vi "Set Steer Motors.vi"(5 "Disable":bool, 6 "PPR":dbl=1024.0, 7 "Offset Encoder Positions":dbl[](array[numeric]), 8 "Steer Control Mode":T2, 9 "Motor List":T1[](array[typedef])=[enum."Right-Front", enum."Left-Front", enum."Left-Back", enum."Right-Back"], 10 "Swerve Data":T8 {"Back Right"."Angle" scale format="%.3f"; "Back Right"."Velocity" scale=-1.0..1.0 scale format="%.1f"; "Back Left"."Angle" scale format="%.3f"; "Back Left"."Velocity" scale=-1.0..1.0 scale format="%.1f"; "Front Left"."Angle" scale format="%.3f"; "Front Left"."Velocity" scale=-1.0..1.0 scale format="%.1f"; "Front Right"."Angle" scale format="%.3f"; "Front Right"."Velocity" scale=-1.0..1.0 scale format="%.1f"}, 11 "Steer Refs":T3[](array[typedef])) -> (1 "Encoder Counts Out":dbl[](array[numeric]), 3 "Array Out":T3[](array[typedef]))   [LabVIEW 2023, in "TShirtWork-SwerveDrive_ACT_ts.lvlib"]
uses:
  TShirtWork-SwerveDrive_ACT_ts.lvlib
  <vilib>/Rock Robotics/WPI/ThirdParty/Phoenix-LabVIEW/Motor Controller/Controls/CTRE_Phoenix_MotorControl_ControlMode.ctl
  Type Defs/ENUM_Steer Mode Select.ctl
  <vilib>/Rock Robotics/SystemInterfaces/DIO/FPGA_DIOPWMChannel.ctl
  <vilib>/Rock Robotics/WPI/PWM/WPI_PWMDeadband.ctl
  <vilib>/Rock Robotics/WPI/MotorControl/WPI_MotorControlType.ctl
  <vilib>/Rock Robotics/SystemInterfaces/DIO/FPGA_DIOChannel.ctl
  <vilib>/Rock Robotics/WPI/MotorControl/WPI_MotorControlDeviceRef.ctl
  Shared Code/TypeDefs/ENUM_Module Position.ctl
  Shared Code/TypeDefs/Level_Velocity plus-minus 1.ctl
  Shared Code/TypeDefs/Dial_Compase heading unit circle CCW positive.ctl
  Shared Code/TypeDefs/Cluster_Module Velocity-Direction-Rotations.ctl
  Shared Code/TypeDefs/Cluster_Swerve 4 Steer and Velocity.ctl
panel:
  # "\"Front\" of Robot"
  # "Right Hand Rule"
  # "X"
  # "+CCW"
  # "Y"
  # "(0,0)"
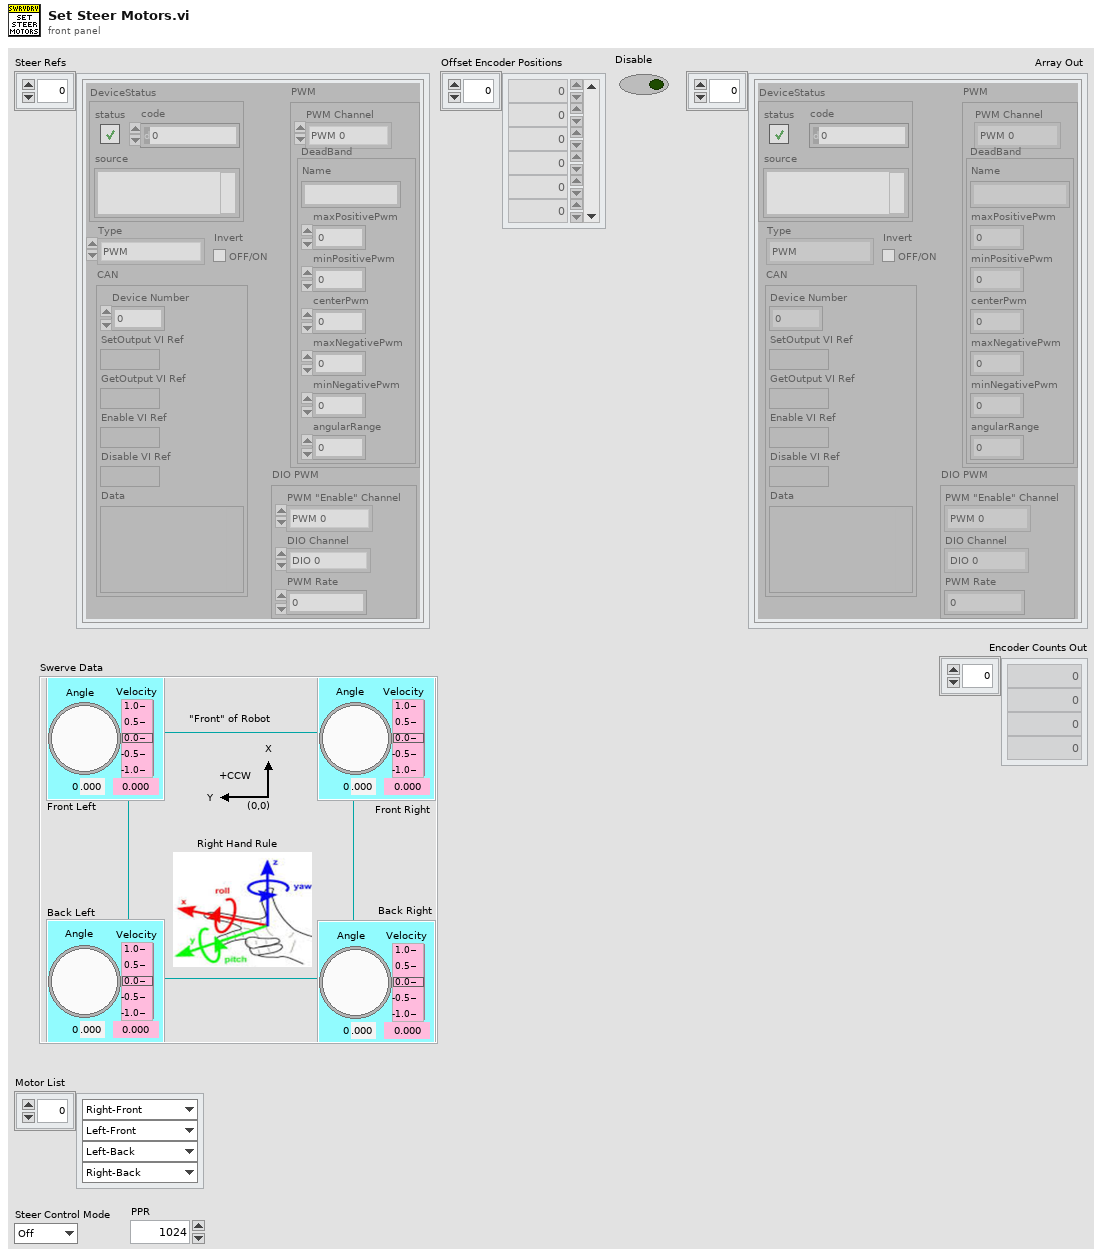
[diagram p1: front panel]
types:
  T1 = typedef "ENUM_Module Position.ctl" = enum16{"Left-Front", "Right-Front", "Left-Back", "Right-Back"}
  T2 = typedef "ENUM_Steer Mode Select.ctl" = enum16{"Off", "Hold", "Steer"}
  T3 = typedef "WPI_MotorControlDeviceRef.ctl" = cluster{"DeviceStatus":errorcluster, "Type":T4, "PWM":cluster{"PWM Channel":T5, "DeadBand":T6}, "CAN":cluster{"Device Number":u8, "SetOutput VI Ref":variant, "GetOutput VI Ref":variant, "Enable VI Ref":variant, "Disable VI Ref":variant, "Data":variant}, "Invert":bool, "DIO PWM":cluster{"PWM \"Enable\" Channel":T5, "DIOChannel":T7, "PWM Rate":dbl}}
  T4 = typedef "WPI_MotorControlType.ctl" = enum16{"PWM", "CAN", "DIO PWM"}
  T5 = typedef "FPGA_DIOPWMChannel.ctl" = enum8{"PWM 0", "PWM 1", "PWM 2", "PWM 3", "PWM 4", "PWM 5", "PWM 6", "PWM 7", "PWM 8", "PWM 9", "PWM MXP 0", "PWM MXP 1", "PWM MXP 2", "PWM MXP 3", "PWM MXP 4", "PWM MXP 5", "PWM MXP 6", "PWM MXP 7", "PWM MXP 8", "PWM MXP 9", "Invalid"}
  T6 = typedef "WPI_PWMDeadband.ctl" = cluster{"Name":string, "maxPositivePwm":i32, "minPositivePwm":i32, "centerPwm":i32, "maxNegativePwm":i32, "minNegativePwm":i32, "angularRange":u16}
  T7 = typedef "FPGA_DIOChannel.ctl" = enum8{"DIO 0", "DIO 1", "DIO 2", "DIO 3", "DIO 4", "DIO 5", "DIO 6", "DIO 7", "DIO 8", "DIO 9", "DIO MXP 0", "DIO MXP 1", "DIO MXP 2", "DIO MXP 3", "DIO MXP 4", "DIO MXP 5", "DIO MXP 6", "DIO MXP 7", "DIO MXP 8", "DIO MXP 9", "DIO MXP 10", "DIO MXP 11", "DIO MXP 12", "DIO MXP 13", "DIO MXP 14", "DIO MXP 15", "SPI Port CS1", "SPI Port CS2", "SPI Port CS3", "SPI Port MISO", "SPI Port MOSI", "Invalid"}
  T8 = typedef "Cluster_Swerve 4 Steer and Velocity.ctl" = cluster{"Front Right":T9, "Front Left":T9, "Back Left":T9, "Back Right":T9}
  T9 = typedef "Cluster_Module Velocity-Direction-Rotations.ctl" = cluster{"Velocity":T10, "Angle":T11, "Rotations Count":dbl}
  T10 = typedef "Level_Velocity plus-minus 1.ctl" = dbl
  T11 = typedef "Dial_Compase heading unit circle CCW positive.ctl" = dbl
  T12 = typedef "CTRE_Phoenix_MotorControl_ControlMode.ctl" = u16
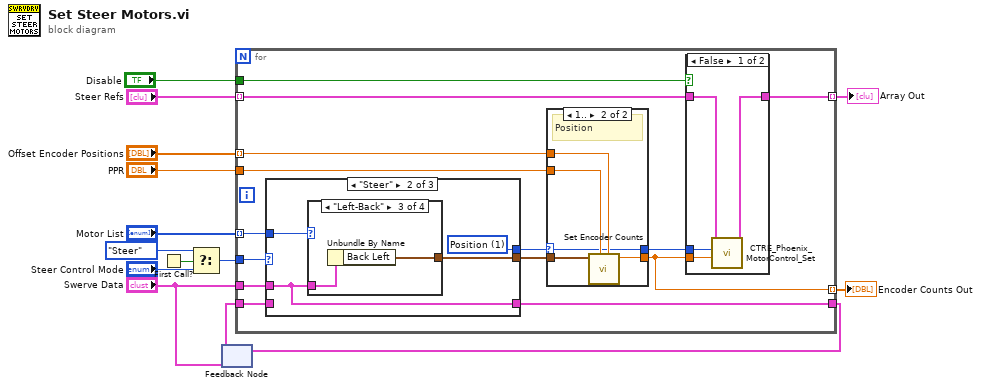
[diagram p0: block diagram]
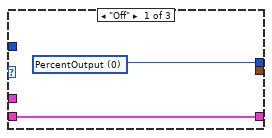
[diagram p3: hidden frame]
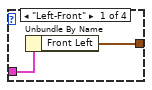
[diagram p4: hidden frame]
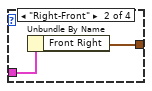
[diagram p5: hidden frame]
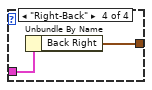
[diagram p6: hidden frame]
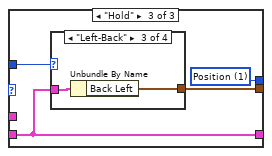
[diagram p7: hidden frame]
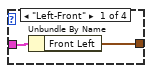
[diagram p8: hidden frame]
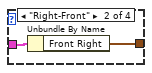
[diagram p9: hidden frame]
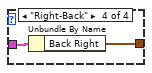
[diagram p10: hidden frame]
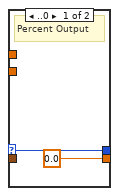
[diagram p11: hidden frame]
diagram:
  n1 = First Call?() -> (First Call?: T/F=w8:bool)
  n2 = Select(t=ENUM_Steer_Mode_Select."Steer" ("Steer Control Mode"), s=w8, f="Steer Control Mode") -> (s? t:f=w5:T2)
  n3 = feedback #1("Swerve Data") -> (w9:T8)
  n4 = for {
    tunnel: "Steer Refs" -> [w28] mode=indexing
    tunnel: "Swerve Data" -> [w25]
    tunnel: [w27] -> w14 mode=indexing
    tunnel: "Offset Encoder Positions" -> [w22] mode=indexing
    tunnel: w5 -> [w26]
    tunnel: "PPR" -> [w23]
    tunnel: "Motor List" -> [w24] mode=indexing
    tunnel: w9 -> [w20]
    tunnel: [w19] -> w3
    tunnel: [w16] -> w2 mode=indexing
    tunnel: "Disable" -> [w15]
    n5 = case shown="\"Steer\"" w26 {
      tunnel: [w35 w39 w51] -> w18
      tunnel: w25 -> [_ w36 _]
      tunnel: w24 -> [_ w38 w50]
      tunnel: [_ w37 w49] -> w21
      tunnel: w20 -> [w34 _ w48]
      tunnel: [w34 w36 w48] -> w19
      frame "Off" {
        w35 = T12 0 items=["PercentOutput"=0, "Position"=1, "Velocity"=2, "Current"=3, "Follower"=5, "MotionProfile"=6, "MotionMagic"=7, "MotionProfileArc"=10, "Disabled"=15] ("Control Mode")
      }
      frame "Steer" {
        w39 = T12 1 items=["PercentOutput"=0, "Position"=1, "Velocity"=2, "Current"=3, "Follower"=5, "MotionProfile"=6, "MotionMagic"=7, "MotionProfileArc"=10, "Disabled"=15] ("Control Mode")
        n6 = case shown="\"Left-Back\"" w38 {
          tunnel: w36 -> [w41 w43 w45 w47]
          tunnel: [w40 w42 w44 w46] -> w37
          frame "Left-Front" {
            n7 = Unbundle By Name(w41) -> ("Front Left"=w40:T9)
          }
          frame "Right-Front" {
            n8 = Unbundle By Name(w43) -> ("Front Right"=w42:T9)
          }
          frame "Left-Back" {
            n9 = Unbundle By Name(w45) -> ("Back Left"=w44:T9)
          }
          frame "Right-Back" {
            n10 = Unbundle By Name(w47) -> ("Back Right"=w46:T9)
          }
        }
      }
      frame "Hold" {
        w51 = T12 1 items=["PercentOutput"=0, "Position"=1, "Velocity"=2, "Current"=3, "Follower"=5, "MotionProfile"=6, "MotionMagic"=7, "MotionProfileArc"=10, "Disabled"=15] ("Control Mode")
        n11 = case shown="\"Left-Back\"" w50 {
          tunnel: w48 -> [w53 w55 w57 w59]
          tunnel: [w52 w54 w56 w58] -> w49
          frame "Left-Front" {
            n12 = Unbundle By Name(w53) -> ("Front Left"=w52:T9)
          }
          frame "Right-Front" {
            n13 = Unbundle By Name(w55) -> ("Front Right"=w54:T9)
          }
          frame "Left-Back" {
            n14 = Unbundle By Name(w57) -> ("Back Left"=w56:T9)
          }
          frame "Right-Back" {
            n15 = Unbundle By Name(w59) -> ("Back Right"=w58:T9)
          }
        }
      }
    }
    n16 = case shown="1.." w18 {
      selector: w18 -> [w60 w62]
      tunnel: w21 -> [_ w65]
      tunnel: w23 -> [_ w64]
      tunnel: w22 -> [_ w63]
      tunnel: [0.0 ("Encder Count Set") w66] -> w16
      tunnel: [w60 w62] -> w17
      frame ..0 {
        # "Percent Output"
      }
      frame 1.. {
        # "Position"
        n17 = call "Set Encoder Counts.vi"("Encoder Count at Zero"=w63, "PPR"=w64, "Angle(0-1) in"=w65) -> ("Encder Count Set"=w66:dbl)  [unwired: 8 in]
      }
    }
    n18 = case shown="False" w15 {
      tunnel: w28 -> [w32 w33]
      tunnel: [w31 w33] -> w27
      tunnel: w17 -> [w30 _]
      tunnel: w16 -> [w29 _]
      frame False {
        n19 = call <vilib>:"CTRE_Phoenix_MotorControl_Set.vi"("Output"=w29, "Control Mode"=w30, "PhoenixMotorControlDevRef"=w32) -> ("PhoenixMotorControlDevRef"=w31:T3)  [unwired: 7 in, 1 out]
      }
      frame True {
      }
    }
  }
  "Array Out" <- w14
  "Encoder Counts Out" <- w2
  n20 = feedback-in #1(w3) -> ()
